vi "REORDER CHECKED IN DATA.vi"(9 "DATA IN":string[][](array[string])) -> (1 "DATA OUT":string[][](array[string]))   [LabVIEW 2019]
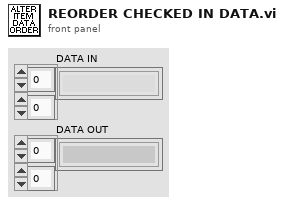
[diagram p1: front panel]
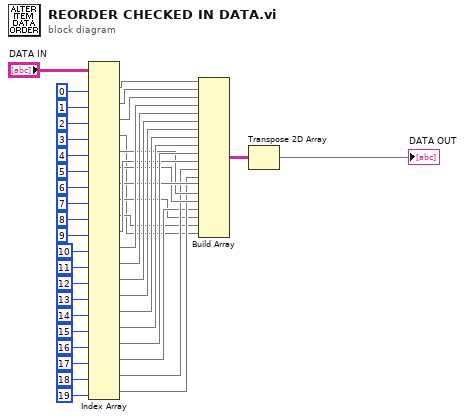
[diagram p0: block diagram]
diagram:
  n1 = Index Array(array="DATA IN", index (col) #1=0 ("index (row)"), index (col) #2=1 ("index (row)"), index (col) #3=2 ("index (row)"), index (col) #4=3 ("index (row)"), index (col) #5=4 ("index (row)"), index (col) #6=5 ("index (row)"), index (col) #7=6 ("index (row)"), index (col) #8=7 ("index (row)"), index (col) #9=8 ("index (row)"), index (col) #10=9 ("index (row)"), index (col) #11=10 ("index (row)"), index (col) #12=11 ("index (row)"), index (col) #13=12 ("index (row)"), index (col) #14=13 ("index (row)"), index (col) #15=14 ("index (row)"), index (col) #16=15 ("index (row)"), index (col) #17=16 ("index (row)"), index (col) #18=17 ("index (row)"), index (col) #19=18 ("index (row)"), index (col) #20=19 ("index (row)")) -> (element #1=w23:string[], element #2=w22:string[], element #3=w21:string[], element #4=w1:string[], element #5=w11:string[], element #6=w10:string[], element #7=w12:string[], element #8=w3:string[], element #9=w2:string[], element #10=w13:string[], element #11=w20:string[], element #12=w19:string[], element #13=w18:string[], element #14=w17:string[], element #15=w16:string[], element #16=w15:string[], element #17=w14:string[], element #18=w4:string[], element #19=w6:string[], element #20=w5:string[])  [unwired: 20 in]
  n2 = Build Array(w23, w22, w21, w20, w19, w18, w17, w16, w15, w14, w13, w6, w5, w12, w11, w10, w4, w3, w2, w1) -> (w9:string[][])
  n3 = Transpose 2D Array(2D array=w9) -> (transposed array=→"DATA OUT":string[][])
